vi "lockchecker.vi"() -> ()   [LabVIEW 2013]
panel:
  out "error out":errorcluster
  in  "error in":errorcluster
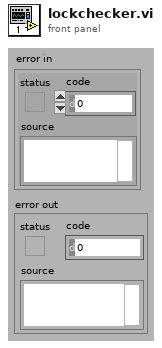
[diagram p1: front panel]
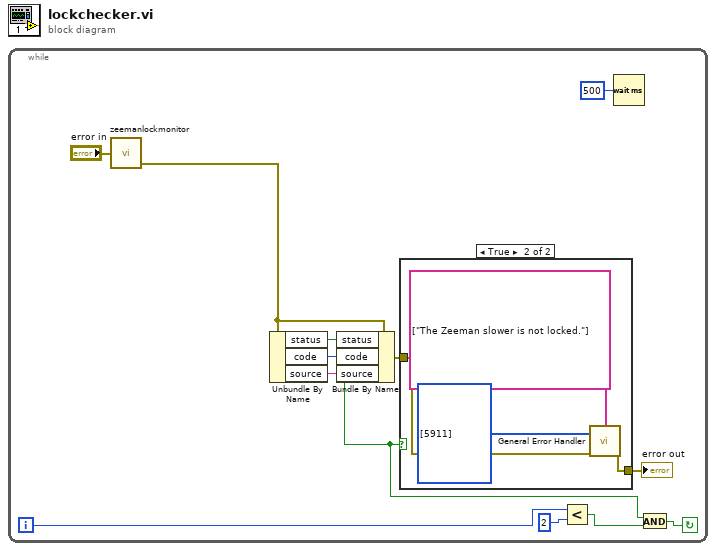
[diagram p0: block diagram]
diagram:
  n1 = while {
    i -> [w8]
    stop <- w11 continue-if-true
    n2 = call "zeemanlockmonitor.vi"("error in"="error in") -> ("error out"=w5:errorcluster)  [unwired: 1 in, 1 out]
    n3 = Unbundle By Name(w5) -> ("status"=w1:bool, "code"=w4:i32, "source"=w3:string)
    n4 = Bundle By Name(cluster=w5, "status"=w1, "code"=w4, "source"=w3) -> (w2:errorcluster)
    n5 = case shown="True" w1 {
      tunnel: [w13 w17] -> w6
      tunnel: w2 -> [w13 w16]
      frame False {
        # "All is well.  Nothing happens."
      }
      frame True {
        n6 = call <vilib>:"General Error Handler.vi"("[user-defined codes]"=i32[] [5911], "[user-defined descriptions]"=string[] ["The Zeeman slower is not locked."], "error in (no error)"=w16) -> ("error out"=w17:errorcluster)  [unwired: 8 in, 4 out]
      }
    }
    "error out" <- w6
    n7 = Less?(x=w8, y=2) -> (x < y?=w10:bool)
    n8 = Wait (ms)(milliseconds to wait=u32 500) -> ()  [unwired: 1 out]
    n9 = And(x=w1, y=w10) -> (x .and. y?=w11:bool)
  }
